vi "Menu Viewer - Add Children.vi"(9 "name":string, 10 "Variant":variant, 11 "TreeControl in":refnum<vi>) -> (1 "Array out":string[](array[string]), 2 "Variant":variant, 3 "TreeControl out":refnum<vi>)   [LabVIEW 2019]
doc: "JSMA Module Template - Top Level UI 0.2.0.4\nRob Humfeld - Jet Engineering\nCopyright (c) 2019, Jet Engineering"
uses:
  private/Button Config Cluster STYP.ctl
  Menu Button.xctl
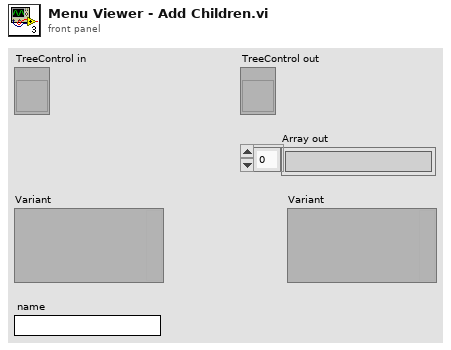
[diagram p1: front panel]
types:
  T1 = typedef "Menu Button.xctl/Button Config Cluster STYP.ctl" = cluster{"ID":string, "Name":string, "Action":string, "Value":string, "Enable?":bool, "Color":string}
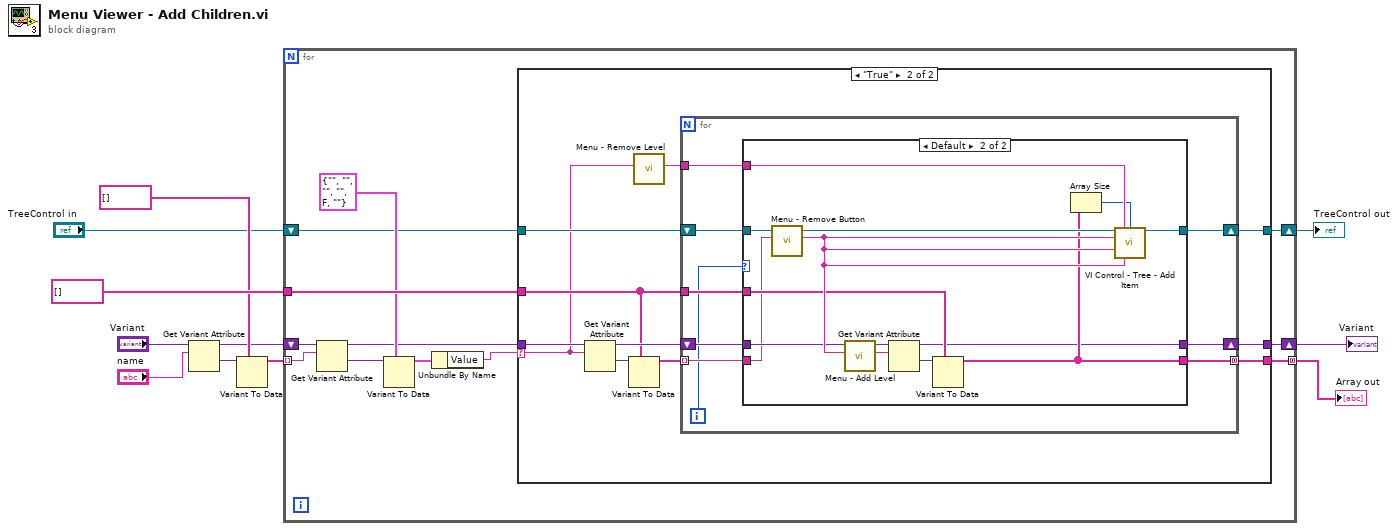
[diagram p0: block diagram]
diagram:
  n1 = Get Variant Attribute(Variant="Variant", name="name") -> (duplicate Variant=w3:variant, value=w5:variant)  [unwired: 2 in, 2 out]
  n2 = Variant To Data(type=string[] [], Variant=w5) -> (data=w2:string[])  [unwired: 1 in, 1 out]
  n3 = for {
    tunnel: [w22] -> w10 mode=concatenating
    tunnel: string[] [] ("Array in") -> [w21]
    shift-right: [w20] -> w8
    shift-left: w3 -> [w16]
    tunnel: w2 -> [w14] mode=indexing
    shift-right: [w23] -> w11
    shift-left: "TreeControl in" -> [w13]
    n4 = Get Variant Attribute(Variant=w16, name=w14) -> (duplicate Variant=w15:variant, value=w12:variant)  [unwired: 2 in, 2 out]
    n5 = Variant To Data(type=T1 {"ID"="", "Name"="", "Action"="", "Value"="", "Enable?"=FALSE, "Color"=""}, Variant=w12) -> (data=w18:T1)  [unwired: 1 in, 1 out]
    n6 = Unbundle By Name(w18) -> ("Value"=w17:string)
    n7 = case shown="\"True\"" w17 {
      selector: w17 -> [_ w26]
      tunnel: [w25 w36] -> w23
      tunnel: [_ w35] -> w22
      tunnel: w13 -> [w25 w30]
      tunnel: w21 -> [_ w29]
      tunnel: [w24 w28] -> w20
      tunnel: w15 -> [w24 w27]
      frame "False", Default {
      }
      frame "True" {
        n8 = Get Variant Attribute(Variant=w27, name=w26) -> (duplicate Variant=w33:variant, value=w31:variant)  [unwired: 2 in, 2 out]
        n9 = Variant To Data(type=w29, Variant=w31) -> (data=w34:string[])  [unwired: 1 in, 1 out]
        n10 = call "Menu - Remove Level.vi"("In"=w26) -> ("Out"=w32:string)  [unwired: 10 in]
        n11 = for {
          tunnel: [w44] -> w35 mode=concatenating
          tunnel: w32 -> [w43]
          tunnel: w29 -> [w41]
          tunnel: w34 -> [w40] mode=indexing
          shift-right: [w38] -> w36
          shift-left: w30 -> [w45]
          shift-right: [w37] -> w28
          shift-left: w33 -> [w42]
          i -> [w39]
          n12 = case shown="Default" w39 {
            tunnel: w45 -> [w47 w58]
            tunnel: w43 -> [_ w57]
            tunnel: w41 -> [_ w53]
            tunnel: [_ w52] -> w44
            tunnel: w42 -> [w46 w51]
            tunnel: w40 -> [_ w50]
            tunnel: [w47 w49] -> w38
            tunnel: [w46 w48] -> w37
            frame 0 {
            }
            frame Default {
              n13 = call "Menu - Remove Button.vi"("In"=w50) -> ("Out"=w55:string)  [unwired: 10 in]
              n14 = call "Menu - Add Level.vi"("In"=w55) -> ("Out"=w54:string)  [unwired: 10 in]
              n15 = Get Variant Attribute(Variant=w51, name=w54) -> (duplicate Variant=w48:variant, value=w59:variant)  [unwired: 2 in, 2 out]
              n16 = Variant To Data(type=w53, Variant=w59) -> (data=w52:string[])  [unwired: 1 in, 1 out]
              n17 = Array Size(array=w52) -> (size(s)=w56:i32)
              n18 = call <userlib>:"VI Control - Tree - Add Item.vi"("Tree.refnum"=w58, "Parent Tag"=w57, "Number of Children"=w56, "ItemTag"=w55, "ItemLabel"=w55, "ItemText"=w55) -> ("Tree.refnum"=w49:refnum<vi>)  [unwired: 7 in, 2 out]
            }
          }
        }
      }
    }
  }
  "TreeControl out" <- w11
  "Array out" <- w10
  "Variant" <- w8
